vi "CursorsDisplay.vi"(0 "Channel Setting 0":T2 {"Meas Range" items=["-0.1 V~+0.1 V"=0.1, "-0.2 V~0.2 V"=0.2, "-0.5 V~+0.5 V"=0.5, "-1 V~+1 V"=1.0, "-2 V~+2 V"=2.0, "-5 V~+5 V"=5.0, "-10 V~+10 V"=10.0]; "Vertical\nPosition (Div)" min=-5.0 max=5.0 step=0.01 scale=-5.0..5.0 scale format="%.2f"; "Scale\n  Volts/Div" scale=0.01..20.0}, 2 "波形图引用句柄":refnum<vi>, 3 "Channel Setting 1":T2 {"Meas Range" items=["-0.1 V~+0.1 V"=0.1, "-0.2 V~0.2 V"=0.2, "-0.5 V~+0.5 V"=0.5, "-1 V~+1 V"=1.0, "-2 V~+2 V"=2.0, "-5 V~+5 V"=5.0, "-10 V~+10 V"=10.0]; "Vertical\nPosition (Div)" min=-5.0 max=5.0 step=0.01 scale=-5.0..5.0 scale format="%.2f"; "Scale\n  Volts/Div" scale=0.01..20.0}, 6 "Cursors":T1 {"CurChan1 2" items=["CH1", "CH2"]; "CurChan1 1" items=["CH1", "CH2"]}, 8 "TriggleSetting":T3={"Type"=enum."Immediate", "Source"="", "Horizontal Position (%)"=2.0, "slope"=10280, "level"=0.0} {"level" format="%0.2f"; "slope" items=["上升"=10280, "下降"=10171]; "Horizontal Position (%)" scale=0.0..1.0}) -> (10 "Cursor":string)   [LabVIEW 2012]
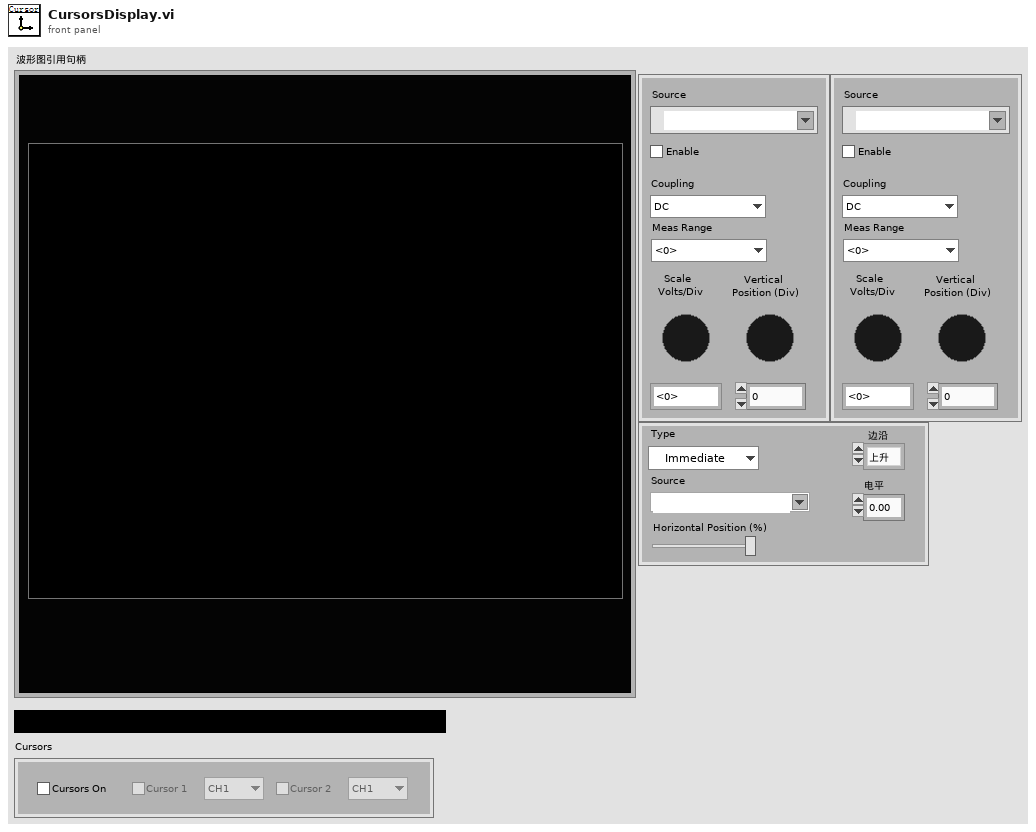
[diagram p1: front panel]
types:
  T1 = cluster{"Cursors On":bool, "Cursor 1":bool, "CurChan1 1":u16, "Cursor 2":bool, "CurChan1 2":u16}
  T2 = cluster{"physical channels":tag, "Enable":bool, "Coupling":enum16{"DC", "AC"}, "    Scale\n  Volts/Div  ":dbl, "    Vertical\nPosition (Div)":dbl, "Meas Range":dbl}
  T3 = cluster{"Type":enum16{"Immediate", "Digital", "Edge"}, "Source":string, "Horizontal Position (%)":dbl, "slope":i32, "level":dbl}
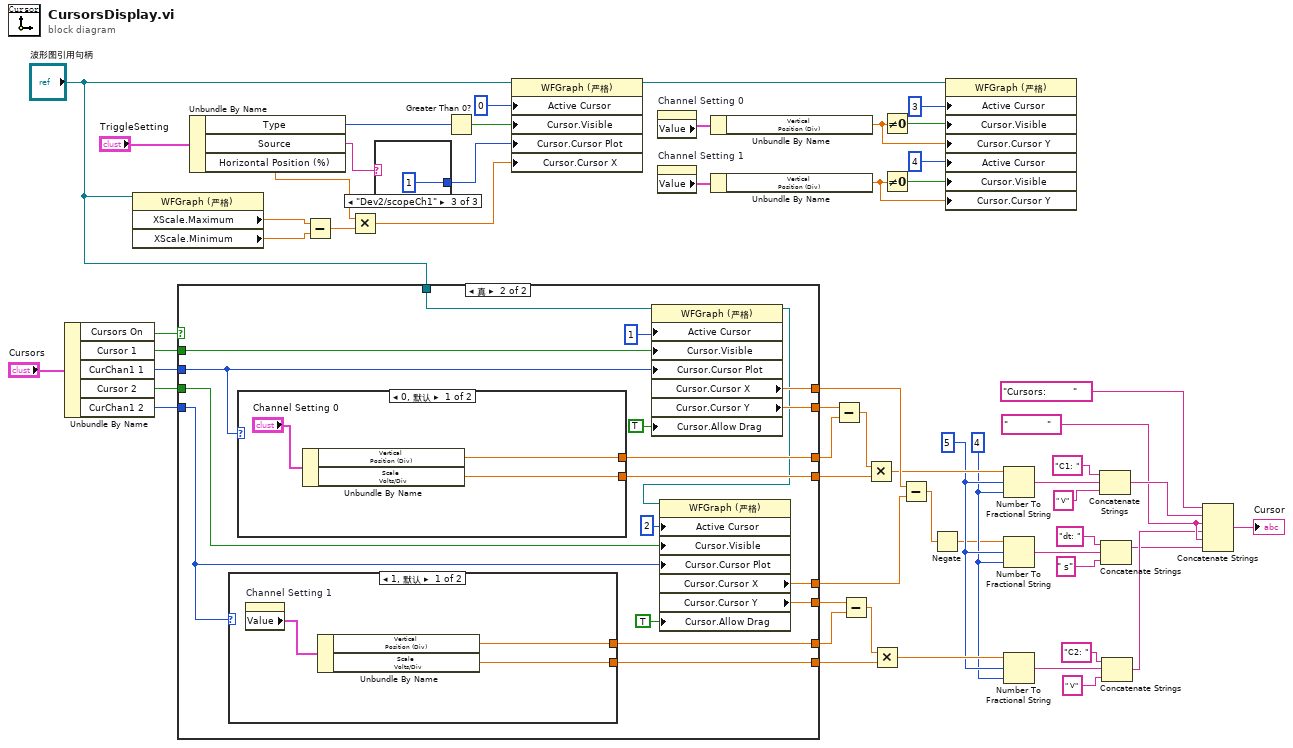
[diagram p0: block diagram]
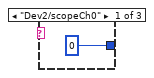
[diagram p2: hidden frame]
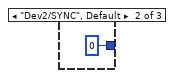
[diagram p3: hidden frame]
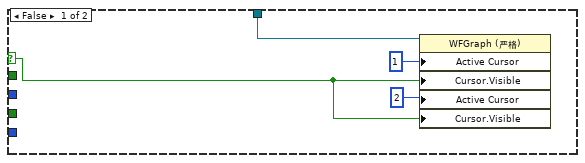
[diagram p4: hidden frame]
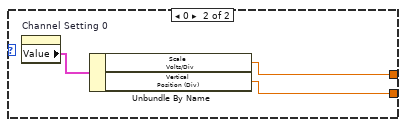
[diagram p5: hidden frame]
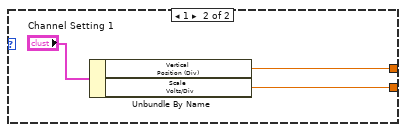
[diagram p6: hidden frame]
diagram:
  w11 = 4
  w26 = 5
  w31 = "             "
  n1 = Unbundle By Name("Cursors") -> ("Cursors On"=w56:bool, "Cursor 1"=w55:bool, "CurChan1 1"=w54:u16, "Cursor 2"=w53:bool, "CurChan1 2"=w52:u16)
  n2 = property class="WFGraph (严格)"(reference="波形图引用句柄") -> ("XScale.Maximum"=w8:dbl, "XScale.Minimum"=w7:dbl)  [unwired: 1 in, 2 out]
  n3 = case shown="真" w56 {
    selector: w56 -> [w59 _]
    tunnel: w55 -> [_ w80]
    tunnel: w54 -> [_ w79]
    tunnel: w53 -> [_ w78]
    tunnel: w52 -> [_ w77]
    tunnel: [_ w76] -> w48
    tunnel: [_ w75] -> w47
    tunnel: [_ w74] -> w44
    tunnel: [_ w73] -> w43
    tunnel: [_ w72] -> w51
    tunnel: [_ w71] -> w50
    tunnel: [_ w70] -> w49
    tunnel: [_ w69] -> w45
    tunnel: "波形图引用句柄" -> [w62 w68]
    frame False {
      n4 = property class="WFGraph (严格)"(reference=w62, "Active Cursor"=u32 1 ("活动游标"), "Cursor.Visible"=w59, "Active Cursor"=u32 2 ("活动游标"), "Cursor.Visible"=w59) -> ()  [unwired: 1 in, 2 out]
    }
    frame True {
      n5 = case shown="1, 默认" w77 {
        tunnel: [w83 w86] -> w74
        tunnel: [w82 w85] -> w73
        frame 1, Default {
          n6 = property on="Channel Setting 1" class="Clust (严格)"() -> ("Value"=w81:T2)  [unwired: 2 in, 2 out]
          n7 = Unbundle By Name(w81) -> ("Vertical\nPosition (Div)"=w83:dbl, "Scale\n  Volts/Div"=w82:dbl)
        }
        frame 0 {
          n8 = property on="Channel Setting 0" class="Clust (严格)"() -> ("Value"=w84:T2)  [unwired: 2 in, 2 out]
          n9 = Unbundle By Name(w84) -> ("Scale\n  Volts/Div"=w86:dbl, "Vertical\nPosition (Div)"=w85:dbl)
        }
      }
      n10 = case shown="0, 默认" w79 {
        tunnel: [w88 w91] -> w76
        tunnel: [w87 w90] -> w75
        frame 0, Default {
          n11 = Unbundle By Name("Channel Setting 0") -> ("Vertical\nPosition (Div)"=w88:dbl, "Scale\n  Volts/Div"=w87:dbl)
        }
        frame 1 {
          n12 = Unbundle By Name("Channel Setting 1") -> ("Vertical\nPosition (Div)"=w91:dbl, "Scale\n  Volts/Div"=w90:dbl)
        }
      }
      n13 = property class="WFGraph (严格)"(reference=w68, "Active Cursor"=u32 1 ("活动游标"), "Cursor.Visible"=w80, "Cursor.Cursor Plot"=w79, "Cursor.Allow Drag"=TRUE ("游标.允许拖曳")) -> (reference out=w65:refnum<vi>, "Cursor.Cursor X"=w72:dbl, "Cursor.Cursor Y"=w70:dbl)  [unwired: 1 in, 1 out]
      n14 = property class="WFGraph (严格)"(reference=w65, "Active Cursor"=u32 2 ("活动游标"), "Cursor.Visible"=w78, "Cursor.Cursor Plot"=w77, "Cursor.Allow Drag"=TRUE ("游标.允许拖曳")) -> ("Cursor.Cursor X"=w71:dbl, "Cursor.Cursor Y"=w69:dbl)  [unwired: 1 in, 2 out]
    }
  }
  n15 = Unbundle By Name("TriggleSetting") -> ("Type"=w57:enum16{"Immediate", "Digital", "Edge"}, "Source"=w6:string, "Horizontal Position (%)"=w3:dbl)
  n16 = Subtract(x=w8, y=w7) -> (x-y=w4:dbl)
  n17 = Multiply(x=w3, y=w4) -> (x*y=w2:dbl)
  n18 = case shown="\"Dev2/scopeCh1\"" w6 {
    tunnel: [0 0 1] -> w5
    frame "Dev2/scopeCh0" {
    }
    frame "Dev2/SYNC", Default {
    }
    frame "Dev2/scopeCh1" {
    }
  }
  n19 = Greater Than 0?(x=w57) -> (x > 0?=w22:bool)
  n20 = property class="WFGraph (严格)"(reference="波形图引用句柄", "Active Cursor"=u32 0 ("活动游标"), "Cursor.Visible"=w22, "Cursor.Cursor Plot"=w5, "Cursor.Cursor X"=w2) -> (reference out=w15:refnum<vi>)  [unwired: 1 in, 1 out]
  n21 = property on="Channel Setting 0" class="Clust (严格)"() -> ("Value"=w13:T2)  [unwired: 2 in, 2 out]
  n22 = property on="Channel Setting 1" class="Clust (严格)"() -> ("Value"=w12:T2)  [unwired: 2 in, 2 out]
  n23 = Unbundle By Name(w13) -> ("Vertical\nPosition (Div)"=w19:dbl)
  n24 = Unbundle By Name(w12) -> ("Vertical\nPosition (Div)"=w16:dbl)
  n25 = Subtract(x=w49, y=w48) -> (x-y=w46:dbl)
  n26 = Subtract(x=w45, y=w44) -> (x-y=w42:dbl)
  n27 = Multiply(x=w46, y=w47) -> (x*y=w41:dbl)
  n28 = Multiply(x=w42, y=w43) -> (x*y=w40:dbl)
  n29 = Not Equal To 0?(x=w19) -> (x != 0?=w20:bool)
  n30 = Not Equal To 0?(x=w16) -> (x != 0?=w17:bool)
  n31 = Subtract(x=w51, y=w50) -> (x-y=w9:dbl)
  n32 = Negate(x=w9) -> (-x=w10:dbl)
  n33 = property class="WFGraph (严格)"(reference=w15, "Active Cursor"=u32 3 ("活动游标"), "Cursor.Visible"=w20, "Cursor.Cursor Y"=w19, "Active Cursor"=u32 4 ("活动游标"), "Cursor.Visible"=w17, "Cursor.Cursor Y"=w16) -> ()  [unwired: 1 in, 2 out]
  n34 = Number To Fractional String(number=w41, width (-)=w26, precision (6)=w11) -> (F-format string=w37:string)  [unwired: 1 in]
  n35 = Number To Fractional String(number=w10, width (-)=w26, precision (6)=w11) -> (F-format string=w38:string)  [unwired: 1 in]
  n36 = Number To Fractional String(number=w40, width (-)=w26, precision (6)=w11) -> (F-format string=w35:string)  [unwired: 1 in]
  n37 = Concatenate Strings("C1: ", w37, " V") -> (w32:string)
  n38 = Concatenate Strings("dt: ", w38, " s") -> (w29:string)
  n39 = Concatenate Strings("C2: ", w35, " V") -> (w30:string)
  n40 = Concatenate Strings("Cursors:         ", w32, w31, w30, w31, w29) -> (→"Cursor":string)
